vi "Run - API Logging (SubVI).vi"(8 "error in (no error)":errorcluster, 10 "Cluster":T1 {"M Event" items=["Stop", "Running", "PID", "Up Limit", "Down Limit", "Load Limit"]; "Test Type" items=["Please Select", "Triaxial Shear", "Triaxial UU", "Shearbox", "Permeability", "Consolidation (Stepped Loading)/Swelling", "Saturation (Incremental)", "User Defined", "UCT", "Isotropic Consolidation", "Swelling Pressure"]; "Data"."Test Type" items=["Please Select", "Triaxial Shear", "Triaxial UU", "Shearbox", "Permeability", "Consolidation (Stepped Loading)/Swelling", "Saturation (Incremental)", "User Defined", "UCT", "Isotropic Consolidation", "Swelling Pressure"]}) -> (0 "error out":errorcluster, 2 "Cluster 2":T1 {"M Event" items=["Stop", "Running", "PID", "Up Limit", "Down Limit", "Load Limit"]; "Test Type" items=["Please Select", "Triaxial Shear", "Triaxial UU", "Shearbox", "Permeability", "Consolidation (Stepped Loading)/Swelling", "Saturation (Incremental)", "User Defined", "UCT", "Isotropic Consolidation", "Swelling Pressure"]; "Data"."Test Type" items=["Please Select", "Triaxial Shear", "Triaxial UU", "Shearbox", "Permeability", "Consolidation (Stepped Loading)/Swelling", "Saturation (Incremental)", "User Defined", "UCT", "Isotropic Consolidation", "Swelling Pressure"]}, 3 "body":string)   [LabVIEW 2019]
uses:
  Controls/RunTest - Data Structure.ctl
  Controls/Test Panel - Data Structure.ctl
  Controls/Station - Test Type.ctl
  <vilib>/Utility/miscctls.llb/LVRowAndColumnTypeDef.ctl
  Controls/RunTest - Calculate Data.ctl
  <vilib>/httpClient/ClientHandle.ctl
  Controls/RunTest - Start Condition.ctl
  Controls/RunTest - Stop Condition.ctl
  Controls/UDP - Event.ctl
  Controls/eFGV States.ctl
  <vilib>/httpClient/POSTBuffer.vi
  <vilib>/httpClient/LabVIEWHTTPClient.lvlib
panel:
  out "Prev Time":dbl
  out "headers":string
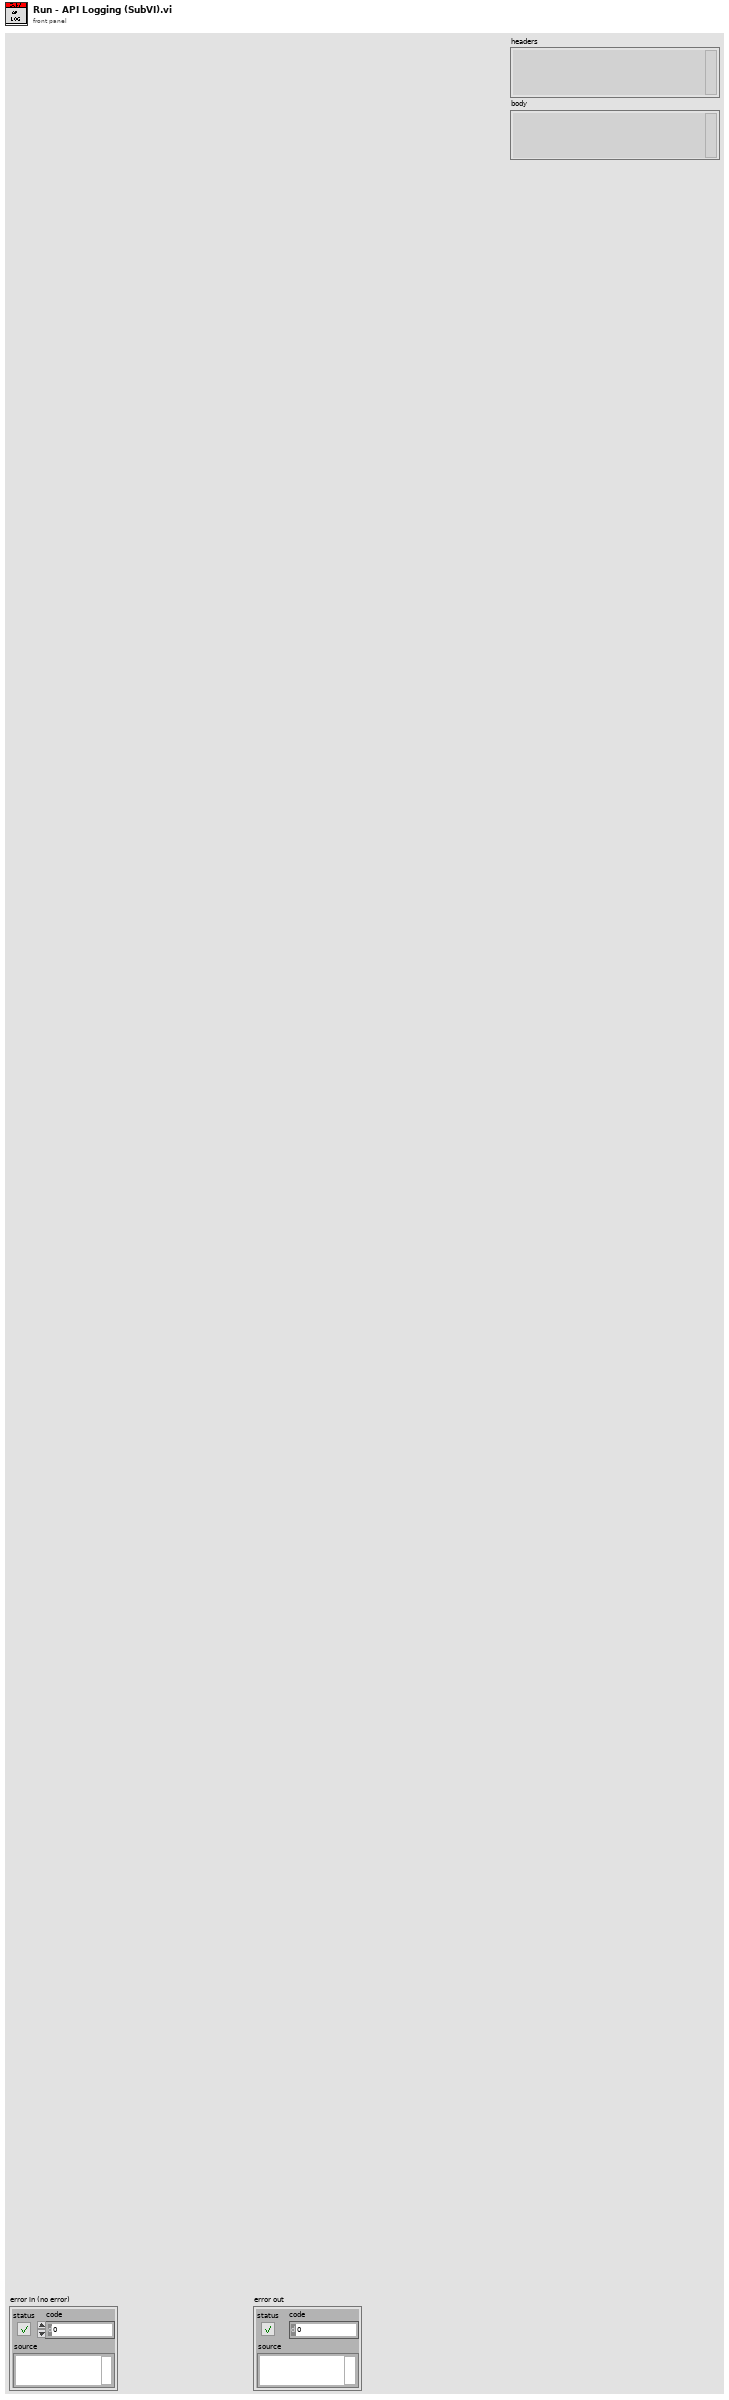
[diagram p1: front panel]
types:
  T1 = typedef "RunTest - Data Structure.ctl" = cluster{"Test Plan":string[], "PlanRow":i32, "Device Name":string[], "Timeout":i32, "Start?":bool, "Pause?":bool, "IP Address":string[], "LogRow":i32, "Logtype":u16, "Log Elapse":sgl, "Data":T2, "Stop log?":bool, "tdms":refnum<k34>, "Sensor Data":sgl[], "Start time":timestamp, "Prev Log Elapse":u32, "Plot":u16, "X-Axis":u16[], "Y-Axis":u16[], "XY":cluster{"X":dbl, "Y":dbl}[][], "End Stage?":bool, "1run":bool, "Condition":u16[], "Start Con":bool, "Log Con":bool, "Stop Con":bool, "Start Elapse":dbl, "Start Load":dbl, "Motor":i32, "StartRow":i32, "number log":i32, "Dir":bool, "Start time test":timestamp, "Auto":bool, "Check return?":bool, "Inv":cluster{"M":i32[], "Bool":bool[]}, "tdms temp":refnum<k34>, "Zero?":bool, "Plot Timer":dbl, "1st Run":bool, "TDMS Path":path, "MaxLoad":dbl, "Log Timer":sgl[], "Test Type":T3, "Log Sensor":string[], "Save?":bool, "1st Log":bool, "Y-Axis 2":u16[], "On Y-Axis 2":bool, "Decimal":u8[], "Init":cluster{"PWP TS":sgl, "Load TS":sgl, "Volume TS":sgl, "Disp TS":sgl, "CP":sgl, "Vol In":sgl, "Vol Out":sgl, "Load UCT":sgl, "Disp UCT":sgl, "PWP Sat":sgl, "CP Sat":sgl, "Volume IsoCons":sgl, "PWP IsoCons":sgl, "PWP TUU":sgl, "Load TUU":sgl, "Volume TUU":sgl, "Disp TUU":sgl, "Load Cons":sgl, "Disp Cons":sgl, "Volume Sat":sgl, "Vertical Load SB":sgl, "Vertical Disp SB":sgl, "H Disp SB":sgl, "H Load SB":sgl}, "Calc":T5, "Device Index":i32[], "Channel Index":i32[], "http ref":T6, "fileid":string, "Step Cons":cluster{"V Stress":sgl, "H Settlement":sgl}, "RunTest":bool, "Graph Last":i32, "Init?":bool, "Datalog":bool[], "Start":T7, "Stop":T8, "Running?":bool, "StartTime":dbl, "Log Prev Time":dbl, "KeyName":string[], "Test RunTime":dbl, "Log Prev Axial":dbl, "M Event":T9[], "Last Log":bool, "popup":bool, "PreStart UU":bool, "PreStart Sat":bool}
  T2 = typedef "Test Panel - Data Structure.ctl" = cluster{"Station":string, "Sample ID":string, "Job No":string, "Job Description":string, "Filename":string, "Test Type":T3, "Speciment No":string, "Depth":string, "Height":string, "Diameter/Length":string, "Weight":string, "Test Parameter":string, "Station[]":string[], "Edit Pos":T4, "Edit Pos Prev":T4, "Area":string, "Path":string}
  T3 = typedef "Station - Test Type.ctl" = u16
  T4 = typedef "LVRowAndColumnTypeDef.ctl" = cluster{"Row":i32, "Column":i32}
  T5 = typedef "RunTest - Calculate Data.ctl" = cluster{"TS":cluster{"Change PWP":sgl, "Change Vol":sgl, "Axial Load":sgl, "CiL":sgl, "Deviator":sgl, "Axial Strain":sgl, "MaxDeviator":sgl}, "TUU":cluster{"Change PWP":sgl, "Axial Load":sgl, "CiL":sgl, "Deviator":sgl, "Axial Strain":sgl, "MaxDeviator":sgl}, "Sat":cluster{"B Value":sgl, "PWP Diss":sgl, "CPP":sgl, "CV":sgl}, "Per":cluster{"Change Vol In":sgl, "Change Vol Out":sgl, "Mean Vol":sgl, "Gradient Pressure":sgl, "Outlet Flow":sgl, "Inlet Flow":sgl, "I X1":sgl, "I X2":sgl, "I Y1":sgl, "I Y2":sgl, "O X1":sgl, "O X2":sgl, "O Y1":sgl, "O Y2":sgl}, "Step Cons":cluster{"V Stress":sgl, "H Settlement":sgl, "Total H Settle":sgl, "Prev Total H":sgl}, "UCT":cluster{"ALC":sgl, "H Change":sgl, "Deviator":sgl, "Axial Strain":sgl, "V Stress":sgl, "MaxDeviator":sgl}, "ISO Cons":cluster{"CPP":sgl, "PWP Diss":sgl, "CV":sgl}, "SB":cluster{"Speci LenC":sgl, "Shear Strain":sgl, "H LC":sgl, "Normal Stress":sgl, "Shear Stress":sgl, "MaxShear":sgl}}
  T6 = typedef "LabVIEWHTTPClient.lvlib/ClientHandle.ctl" = refnum<k1>
  T7 = typedef "RunTest - Start Condition.ctl" = cluster{"Cons":cluster{"VS":dbl, "Delay":bool, "No Delay":dbl}, "Sat":cluster{"CP":dbl, "BP":dbl, "StartBP":bool, "Target CP":bool, "Target BP":bool}, "Iso":cluster{"BP":dbl}, "TS":cluster{"SS":dbl, "Engage":bool, "ES":dbl, "LC":dbl, "PreStart":bool, "Trig SS":bool, "Drain":dbl}, "TUU":cluster{"SS":dbl, "Engage":bool, "ES":dbl, "LC":dbl, "PreStart":bool, "Trig SS":bool, "CP":dbl, "Delay Value":dbl, "Delay":bool, "CP PID":bool}, "UCT":cluster{"SS":dbl, "Engage":bool, "ES":dbl, "LC":dbl, "PreStart":bool, "Trig SS":bool}, "Enable?":bool, "SB":cluster{"SS":dbl, "Engage":bool, "ES":dbl, "LC":dbl, "PreStart":bool, "Trig SS":bool, "VS":dbl, "Delay Value":dbl, "Delay":bool, "VS PID":bool}, "Perm":cluster{"DP":dbl}}
  T8 = typedef "RunTest - Stop Condition.ctl" = cluster{"Cons":cluster{"Select":i32, "Disp":dbl, "Time":dbl, "Time2":dbl, "Disp 2":dbl, "Time Cond":dbl, "Last Disp":dbl, "Swell":bool}, "Sat":cluster{"Select":i32, "PP":dbl, "Time":dbl, "VC":dbl, "Time2":dbl, "Time Cond":dbl, "Last PP":dbl, ".B":bool, "B":dbl, "Last Vc":dbl, "Time Cond 2":dbl, "Time3":dbl, "Time Cond 3":dbl}, "Iso":cluster{"PP":dbl, "Time":dbl, "VC":dbl, "Time2":dbl, "Time Cond":dbl, "Last Vc":dbl, ".PP":bool, "Time Cond 2":dbl, "Select":i32}, "TS":cluster{"Axial":dbl, ".MaxDev":bool, "MaxDev Value":dbl, "Return":bool, "Reset":bool, "Prev Time":dbl, "PostStop Run":bool, "CP Stop":bool, "BP Stop":bool, "PostStop Trig":bool, "Reset Value":dbl, "BPTrig":bool, "CPTrig":bool, "VLCTrig":bool}, "TUU":cluster{"Axial":dbl, ".MaxDev":bool, "MaxDev Value":dbl, "Return":bool, "Reset":bool, "Prev Time":dbl, "PostStop Run":bool, "CP Stop":bool, "BP Stop":bool, "PostStop Trig":bool, "Reset Value":dbl, "BPTrig":bool, "CPTrig":bool, "VLCTrig":bool}, "UCT":cluster{"Axial":dbl, ".MaxDev":bool, "MaxDev Value":dbl, "Return":bool, "Reset":bool, "Prev Time":dbl, "PostStop Run":bool, "CP Stop":bool, "BP Stop":bool, "PostStop Trig":bool}, "Enable?":bool, "SB":cluster{"Shear":dbl, ".MaxShear":bool, "MaxShear Value":dbl, "Return":bool, "Reset":bool, "Prev Time":dbl, "PostStop Run":bool, "CP Stop":bool, "BP Stop":bool, "PostStop Trig":bool, "Reset Value":dbl, "BPTrig":bool, "CPTrig":bool, "VLCTrig":bool}, "Perm":cluster{"Max Time":bool, "Reset":bool, "PostStop Run":bool, "Ratio":bool, "Reset Value":dbl, "Time":dbl, "RatioTime":dbl, "RatioMore":dbl, "RatioLess":dbl, "Time Cond":dbl, "Time Cond 2":dbl, "Prev IF":dbl, "Prev OF":dbl, "PostStop Trig":bool, "BP Trig":bool, "DP Stop":bool, "BP Stop":bool, "CP Stop":bool, "CP Trig":bool}, "SP":cluster{".Max Time":bool, ".Time":bool, "Time":dbl, "MaxTime":dbl, "Time Cond":dbl, "Max Time Cond":dbl, "Stress":dbl}}
  T9 = typedef "UDP - Event.ctl" = u16
  T10 = cluster{"timestamp":string, "elapsetime":string, "testname":string, "testtype":u16, "data":string[], "fileid":string, "stage":string}
  T11 = typedef "eFGV States.ctl" = enum16{"Init", "Read", "Write", "Exit"}
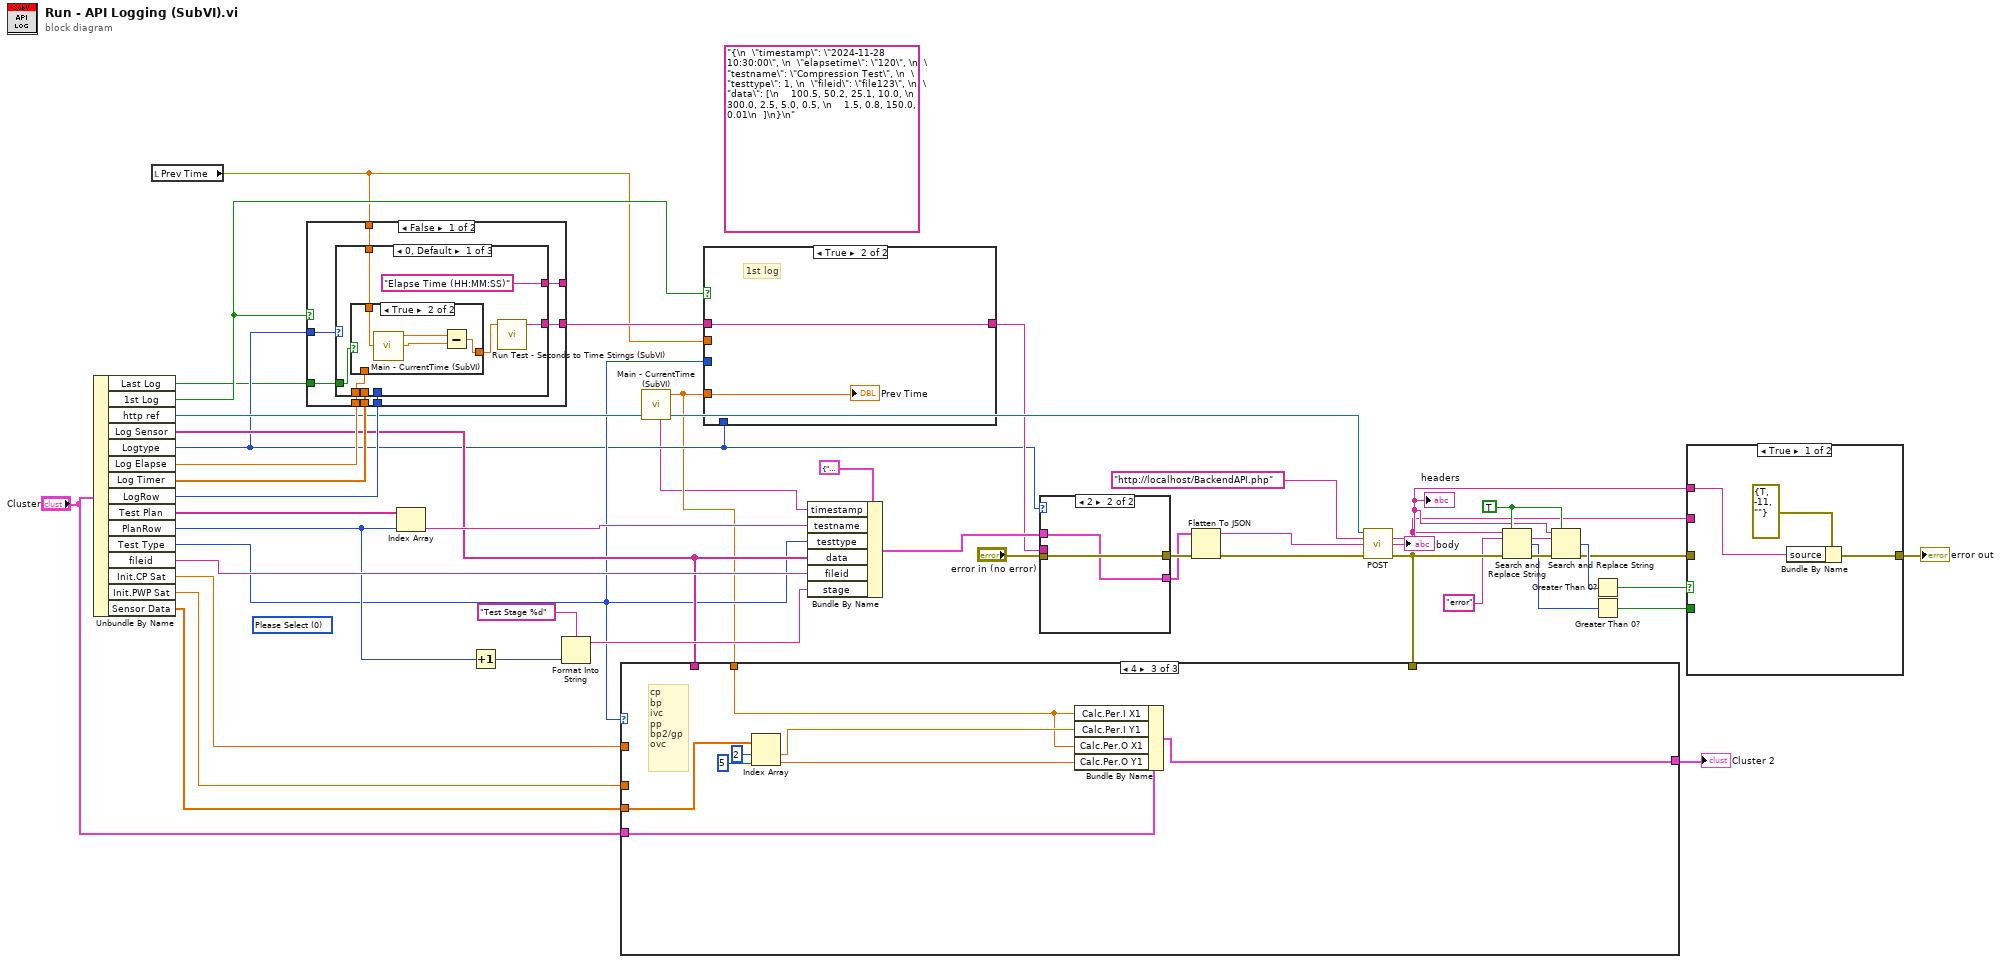
[diagram p0: block diagram]
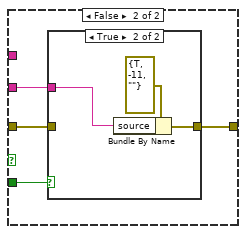
[diagram p2: hidden frame]
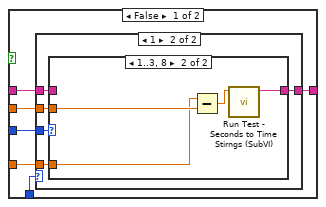
[diagram p4: hidden frame]
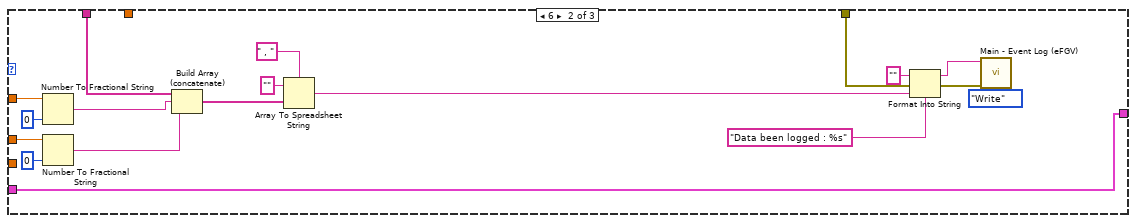
[diagram p8: hidden frame]
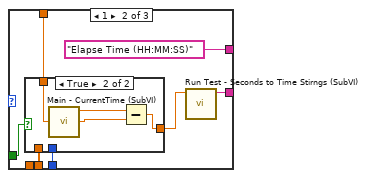
[diagram p10: hidden frame]
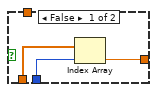
[diagram p11: hidden frame]
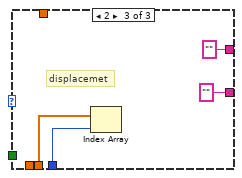
[diagram p12: hidden frame]
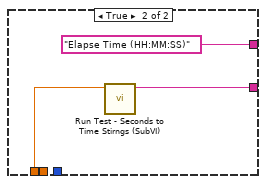
[diagram p13: hidden frame]
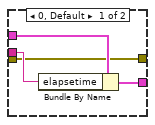
[diagram p14: hidden frame]
diagram:
  w9 = TRUE ("replace all? (F)")
  w12 = "error"
  (unwired) T3 0 items=["Please Select", "Triaxial Shear", "Triaxial UU", "Shearbox", "Permeability", "Consolidation (Stepped Loading)/Swelling", "Saturation (Incremental)", "User Defined", "UCT", "Isotropic Consolidation"] ("Test Type")
  (unwired) "{\n  \"timestamp\": \"2024-11-28 10:30:00\", \n  \"elapsetime\": \"120\", \n  \"testname\": \"Compression Test\", \n  \"testtype\": 1, \n  \"fileid\": \"file123\", \n  \"data\": [\n    100.5, 50.2, 25.1, 10.0, \n    300.0, 2.5, 5.0, 0.5, \n    1.5, 0.8, 150.0, 0.01\n  ]\n}\n"
  n1 = Unbundle By Name("Cluster") -> ("Last Log"=w2:bool, "1st Log"=w15:bool, "http ref"=w33:T6, "Log Sensor"=w27:string[], "Logtype"=w21:u16, "Log Elapse"=w45:sgl, "Log Timer"=w46:sgl[], "LogRow"=w44:i32, "Test Plan"=w43:string[], "PlanRow"=w30:i32, "Test Type"=w24:T3, "fileid"=w32:string, "Init.CP Sat"=w26:sgl, "Init.PWP Sat"=w25:sgl, "Sensor Data"=w20:sgl[])
  n2 = local read "Prev Time"() -> (w1:dbl)
  n3 = case shown="False" w15 {
    tunnel: w46 -> [w54 _]
    tunnel: w44 -> [w53 _]
    tunnel: w45 -> [w52 w84]
    tunnel: w21 -> [w51 _]
    tunnel: [w50 "Elapse Time (HH:MM:SS)" ("String")] -> _
    tunnel: [w49 w82] -> w22
    tunnel: w2 -> [w48 _]
    tunnel: w1 -> [w47 _]
    frame False {
      n4 = case shown="0, Default" w51 {
        tunnel: w54 -> [_ w71 w81]
        tunnel: w53 -> [_ w70 w80]
        tunnel: w52 -> [w57 _ _]
        tunnel: ["Elapse Time (HH:MM:SS)" ("String") "Elapse Time (HH:MM:SS)" ("String") "" ("String")] -> w50
        tunnel: [w59 w67 ""] -> w49
        tunnel: w48 -> [w55 w66 _]
        tunnel: w47 -> [w58 w65 _]
        frame 0, Default {
          n5 = case shown="True" w55 {
            tunnel: w57 -> [w61 _]
            tunnel: [w61 w62] -> w56
            tunnel: w58 -> [_ w63]
            frame False {
            }
            frame True {
              n6 = call "Main - CurrentTime (SubVI).vi"() -> ("Seconds"=w64:dbl)  [unwired: 10 in, 1 out]
              n7 = Subtract(x=w64, y=w63) -> (x-y=w62:dbl)
            }
          }
          n8 = call "Run Test - Seconds to Time Stirngs (SubVI).vi"("Seconds"=w56) -> ("Time Strings"=w59:string)  [unwired: 10 in]
        }
        frame 1 {
          n9 = case shown="True" w66 {
            tunnel: w71 -> [w74 _]
            tunnel: w70 -> [w73 _]
            tunnel: [w72 w75] -> w68
            tunnel: w65 -> [_ w76]
            frame False {
              n10 = Index Array(array=w74, index=w73) -> (element=w72:sgl)
            }
            frame True {
              n11 = call "Main - CurrentTime (SubVI).vi"() -> ("Seconds"=w77:dbl)  [unwired: 10 in, 1 out]
              n12 = Subtract(x=w77, y=w76) -> (x-y=w75:dbl)
            }
          }
          n13 = call "Run Test - Seconds to Time Stirngs (SubVI).vi"("Seconds"=w68) -> ("Time Strings"=w67:string)  [unwired: 10 in]
        }
        frame 2 {
          # "displacemet"
          n14 = Index Array(array=w81, index=w80) -> ()  [unwired: 1 out]
        }
      }
    }
    frame True {
      n15 = call "Run Test - Seconds to Time Stirngs (SubVI).vi"("Seconds"=w84) -> ("Time Strings"=w82:string)  [unwired: 10 in]
    }
  }
  n16 = Index Array(array=w43, index=w30) -> (element=w38:string)
  n17 = Increment(x=w30) -> (x+1=w29:i32)
  n18 = Format Into String(format string="Test Stage %d", w29) -> (resulting string=w28:string)  [unwired: 2 in, 1 out]
  n19 = call "Main - CurrentTime (SubVI).vi"() -> ("Seconds"=w17:dbl, "Time"=w16:string)  [unwired: 10 in]
  n20 = case shown="True" w15 {
    tunnel: w17 -> [w90 w102]
    tunnel: w24 -> [w89 _]
    tunnel: [w88 w103] -> w23
    tunnel: w22 -> [w87 w103]
    tunnel: w1 -> [w86 _]
    tunnel: w21 -> [w85 _]
    frame False {
      n21 = case shown="1" w85 {
        tunnel: w90 -> [_ w96]
        tunnel: w89 -> [_ w95]
        tunnel: [w91 w94] -> w88
        tunnel: w87 -> [w91 w93]
        tunnel: w86 -> [_ w92]
        frame 0, Default {
        }
        frame 1 {
          n22 = case shown="1..3, 8" w95 {
            tunnel: w96 -> [_ w98]
            tunnel: [w97 w99] -> w94
            tunnel: w93 -> [w97 _]
            tunnel: w92 -> [_ w101]
            frame 0, Default {
            }
            frame 1..3, 8 {
              n23 = Subtract(x=w98, y=w101) -> (x-y=w100:dbl)
              n24 = call "Run Test - Seconds to Time Stirngs (SubVI).vi"("Seconds"=w100) -> ("Time Strings"=w99:string)  [unwired: 10 in]
            }
          }
        }
      }
    }
    frame True {
      # "1st log"
      "Prev Time" <- w102
    }
  }
  n25 = Bundle By Name(cluster=T10 {"timestamp"="", "elapsetime"="", "testname"="", "testtype"=0, "data"=[], "fileid"="", "stage"=""}, "timestamp"=w16, "testname"=w38, "testtype"=w24, "data"=w27, "fileid"=w32, "stage"=w28) -> (w39:T10)
  n26 = case shown="2" w21 {
    tunnel: "error in (no error)" -> [w104 w109]
    tunnel: [w104 w109] -> w36
    tunnel: w23 -> [w107 _]
    tunnel: w39 -> [w106 w108]
    tunnel: [w105 w108] -> w35
    frame 0, Default {
      n27 = Bundle By Name(cluster=w106, "elapsetime"=w107) -> (w105:T10)
    }
    frame 2 {
    }
  }
  n28 = Flatten To JSON(anything=w35, error in (no error)=w36) -> (JSON string=w41:string, 11:w34:errorcluster)  [unwired: 1 in]
  n29 = call-poly <vilib>:"POST.vi"("client handle"=w33, "url"="http://localhost/BackendAPI.php", "buffer"=w41, "error in (no error)"=w34) -> ("headers"=w6:string, "body"=w3:string, "error out"=w14:errorcluster)  [unwired: 8 in, 1 out]
  "headers" <- w6
  "body" <- w3
  n30 = case shown="4" w24 {
    tunnel: w27 -> [_ w123 _]
    tunnel: w26 -> [_ w122 _]
    tunnel: w25 -> [_ w119 _]
    tunnel: w14 -> [_ w113 _]
    tunnel: w20 -> [_ _ w136]
    tunnel: "Cluster" -> [w110 w111 w133]
    tunnel: w17 -> [_ _ w130]
    tunnel: [w110 w111 w131] -> w18
    frame 0, Default {
    }
    frame 6 {
      n31 = Number To Fractional String(number=w122, precision (6)=i16 0) -> (F-format string=w118:string)  [unwired: 2 in]
      n32 = Number To Fractional String(number=w119, precision (6)=i16 0) -> (F-format string=w117:string)  [unwired: 2 in]
      n33 = Build Array (concatenate)(w123, w118, w117) -> (w116:string[])
      n34 = Array To Spreadsheet String(delimiter (Tab)=" , ", array=w116, 3:"" ("format string")) -> (spreadsheet string=w114:string)
      n35 = Format Into String(format string="Data been logged : %s", initial string="", error in=w113, w114) -> (resulting string=w126:string, error out=w127:errorcluster)
      n36 = call "Main - Event Log (eFGV).vi"("Action"=eFGV_States."Write", "error in"=w127, "Data In"=w126) -> ()  [unwired: 5 in, 4 out]
    }
    frame 4 {
      # "cp\nbp\nivc\npp\nbp2/gp\novc"
      n37 = Index Array(array=w136, index #1=2 ("index"), index #2=5 ("index")) -> (element #1=w132:sgl, element #2=w129:sgl)
      n38 = Bundle By Name(cluster=w133, "Calc.Per.I X1"=w130, "Calc.Per.I Y1"=w132, "Calc.Per.O X1"=w130, "Calc.Per.O Y1"=w129) -> (w131:T1)
    }
  }
  "Cluster 2" <- w18
  n39 = Search and Replace String(replace all?=w9, input string=w3, search string=w12, error in=w14) -> (number of replacements=w11:i32, error out=w13:errorcluster)  [unwired: 4 in, 2 out]
  n40 = Search and Replace String(replace all?=w9, input string=w6, search string=w12, error in=w13) -> (number of replacements=w10:i32, error out=w7:errorcluster)  [unwired: 4 in, 2 out]
  n41 = Greater Than 0?(x=w10) -> (x > 0?=w8:bool)
  n42 = Greater Than 0?(x=w11) -> (x > 0?=w4:bool)
  n43 = case shown="True" w8 {
    tunnel: w7 -> [_ w140]
    tunnel: w6 -> [w138 _]
    tunnel: [w137 w143] -> w5
    tunnel: w4 -> [_ w142]
    tunnel: w3 -> [_ w141]
    frame True {
      n44 = Bundle By Name(cluster=errorcluster {"status"=TRUE, "code"=-11, "source"=""} ("error out"), "source"=w138) -> (w137:errorcluster)
    }
    frame False {
      n45 = case shown="True" w142 {
        tunnel: w141 -> [_ w146]
        tunnel: [w144 w145] -> w143
        tunnel: w140 -> [w144 _]
        frame False {
        }
        frame True {
          n46 = Bundle By Name(cluster=errorcluster {"status"=TRUE, "code"=-11, "source"=""} ("error out"), "source"=w146) -> (w145:errorcluster)
        }
      }
    }
  }
  "error out" <- w5
